vi "NOSAMSBouncerDAQold.vi"(8 "error in (no error)":errorcluster) -> (0 "error out":errorcluster, 2 "Summary Data":T3={"C12LE"=-3.412199553742333e-06, "C13LE"=5.20479903681381e-07, "C12"=7.075321622517488e-06, "C13L"=1.7362857861361653e-07, "C13H"=-1.0439441090572094e-07, "C1312"=0.009791956480809522, "Counts"=421, "LT"=47.557759786666665, "RT"=50.97312722666666, "BadBlocks"=0} {"C12LE" format="%_3e"; "C13LE" format="%_3e"; "C1312" format="%_3e"; "C12" format="%_3e"; "C13L" format="%_3e"; "C13H" format="%_3e"}, 3 "Run Average Ratios":T7={"C14Rate"=8.852393424091265, "CountErr"=0.04873701788285794, "DT"=3.415367439999997, "DTfrac"=0.06700329420269986, "C13"=144076303000.13074, "C13H/L"=-0.601251313230148, "d13C"=-128.61242295148944, "C14/13"=6.144239711705561e-11, "C12Cor"=14723744296458.893, "C13/12"=0.009791956480809522, "C14/12"=6.012324885471077e-13, "LEC13/12"=-0.15253501311508708} {"LEC13/12" format="%_4e"; "DTfrac" format="%#_3g"; "DT" format="%#_3g"; "CountErr" format="%#_3g"; "d13C" format="%_4g"; "C13/12" format="%_4e"; "C14/12" format="%_4e"; "C14/13" format="%_3e"; "C12Cor" format="%_3e"; "C13" format="%_3e"; "C13H/L" format="%#_3g"})   [LabVIEW 2011]
uses:
  RunRatios.ctl
  SummaryData.ctl
  PixieKeithleyDAQstates.ctl
  FCOffset.ctl
  BouncerParameters.ctl
  <vilib>/DAQmx/write.llb/DAQmx Write (Analog Wfm 1Chan NSamp).vi
  <vilib>/DAQmx/read.llb/DAQmx Read (Analog 1D Wfm NChan NSamp).vi
  <vilib>/DAQmx/read.llb/DAQmx Read (Counter U32 1Chan 1Samp).vi
  <vilib>/DAQmx/create/channels.llb/DAQmx Create Channel (CI-Count Edges).vi
  <vilib>/DAQmx/create/channels.llb/DAQmx Create Channel (AI-Voltage-Basic).vi
  <vilib>/DAQmx/configure/trigger.llb/DAQmx Start Trigger (Digital Edge).vi
  <vilib>/DAQmx/configure/timing.llb/DAQmx Timing (Sample Clock).vi
  <vilib>/DAQmx/create/channels.llb/DAQmx Create Channel (AO-Voltage-Basic).vi
  <vilib>/DAQmx/configure/timing.llb/DAQmx Timing (Use Waveform).vi
  <vilib>/DAQmx/create/channels.llb/DAQmx Create Channel (CO-Pulse Generation-Time).vi
  <vilib>/DAQmx/configure/timing.llb/DAQmx Timing (Implicit).vi
  <vilib>/DAQmx/miscellaneous.llb/DAQmx Fill In Error Info.vi
  Program Files/National Instruments/LabVIEW 2011/resource/objmgr/daqmx.rc
panel:
  out "Transmission":dbl format="%#_3g"
  out "C13":dbl
  out "DT Corrected Rate Ch0":dbl=8.852393424091265
  in  "Bouncer Parameters":T1={"12C Period"=0.6, "12C Delay"=400.0, "12C Voltage"=8.264999999999993, "13C Period"=0.6, "13C Delay"=200.0, "13C Voltage"=3.9999999999999996, "14C Period"=100.0, "14C Delay"=800.0, "14C Voltage"=0.41, "LE13C Period"=0.10000000000000003, "LE13C Delay"=100.0, "LE13C Voltage"=0.41, "LE12C Period"=0.20000000000000004, "LE12C Delay"=100.0, "LE12C Voltage"=4.3} {"LE12C Voltage" format="%_4f"; "LE13C Voltage" format="%_4f"; "14C Voltage" format="%_4f"; "13C Voltage" format="%_4f"; "12C Voltage" format="%_4f"}
  out "Split Cup Good":bool
  out "GetBlocktime":dbl
  out "HE 13 Ratio":waveform(dbl)(graph)={"t0"=timestamp(3425919338.3191624 s since 1904-01-01), "dt"=9.999999999999972e-06, "Y"=array[400 elements], "attributes"=variant("NI_ChannelName"=variant(string "PXI1Slot4/ai2"), "NI_UnitDescription"=variant(string "Volts"))}
  out "HE 13 SUM":waveform(dbl)(graph)={"t0"=timestamp(3425919338.3191624 s since 1904-01-01), "dt"=9.999999999999972e-06, "Y"=array[400 elements], "attributes"=variant("NI_ChannelName"=variant(string "PXI1Slot4/ai2"), "NI_UnitDescription"=variant(string "Volts"))}
  in  "low limit":dbl=1e-08
  in  "C13HLPoints":i32=10
  out "LE Currents":cluster{"C13LE":dbl, "C12LE":dbl}(graph)={"C13LE"=0.5227394525948715, "C12LE"=-3.4827548280142357}
  in  "C12":dbl=10000000.0
  in  "C13":dbl=1000000000.0
  in  "C13LE":dbl=1000000.0
  in  "C12LE":dbl=1000000.0
  out "LoopTime":u32=56
  in  "AI rate":dbl=100000.0 format="%0.2f"
  in  "AI Samples":i32=1000
  out "CH1 GDT":dbl=3.2435650133333334
  out "CH0 GDT":dbl=3.2435607466666667
  in  "FC Offset":T2={"HE 12C Offset"=0.0, "HE 13CL Offset"=0.0, "HE 13CH Offset"=0.0, "LE FC Scale"=11, "HE C12 Scale"=11, "HE C13 Scale"=18} {"HE C13 Scale" items=["500 mA/V", "200 mA/V", "100 mA/V", "50 mA/V", "20 mA/V", "10 mA/V", "5 mA/V", "2 mA/V", "1 mA/V", "500 uA/V", "200 uA/V", "100 uA/V", "50 uA/V", "20 uA/V", "10 uA/V", "5 uA/V", "2 uA/V", "1 uA/V", "500 nA/V", "200 nA/V", "100 nA/V", "50 nA/V", "20 nA/V", "10 nA/V", "5 nA/V", "2 nA/V", "1 nA/V", "500 pA/V", "200 pA/V", "100 pA/V", "50 pA/V", "20 pA/V", "10 pA/V", "5 pA/V", "2 pA/V", "1 pA/V", ""]; "HE C12 Scale" items=["500 mA/V", "200 mA/V", "100 mA/V", "50 mA/V", "20 mA/V", "10 mA/V", "5 mA/V", "2 mA/V", "1 mA/V", "500 uA/V", "200 uA/V", "100 uA/V", "50 uA/V", "20 uA/V", "10 uA/V", "5 uA/V", "2 uA/V", "1 uA/V", "500 nA/V", "200 nA/V", "100 nA/V", "50 nA/V", "20 nA/V", "10 nA/V", "5 nA/V", "2 nA/V", "1 nA/V", "500 pA/V", "200 pA/V", "100 pA/V", "50 pA/V", "20 pA/V", "10 pA/V", "5 pA/V", "2 pA/V", "1 pA/V", ""]; "LE FC Scale" items=["500 mA/V", "200 mA/V", "100 mA/V", "50 mA/V", "20 mA/V", "10 mA/V", "5 mA/V", "2 mA/V", "1 mA/V", "500 uA/V", "200 uA/V", "100 uA/V", "50 uA/V", "20 uA/V", "10 uA/V", "5 uA/V", "2 uA/V", "1 uA/V", "500 nA/V", "200 nA/V", "100 nA/V", "50 nA/V", "20 nA/V", "10 nA/V", "5 nA/V", "2 nA/V", "1 nA/V", "500 pA/V", "200 pA/V", "100 pA/V", "50 pA/V", "20 pA/V", "10 pA/V", "5 pA/V", "2 pA/V", "1 pA/V", ""]; "HE 13CH Offset" format="%.1e"; "HE 13CL Offset" format="%_2e"; "HE 12C Offset" format="%_2e"}
  out "HE 13CL Cup":waveform(dbl)(graph)={"t0"=timestamp(3425919338.3191624 s since 1904-01-01), "dt"=9.999999999999972e-06, "Y"=array[400 elements], "attributes"=variant("NI_ChannelName"=variant(string "PXI1Slot4/ai2"), "NI_UnitDescription"=variant(string "Volts"))}
  out "Bouncer":waveform(dbl)(graph)={"t0"=timestamp(3425919338.3171663 s since 1904-01-01), "dt"=9.999999999999972e-06, "Y"=array[1000 elements], "attributes"=variant("NI_ChannelName"=variant(string "PXI1Slot4/ai4"), "NI_UnitDescription"=variant(string "Volts"))}
  out "LE 13C Cup":waveform(dbl)(graph)={"t0"=timestamp(3425919338.3231645 s since 1904-01-01), "dt"=9.999999999999972e-06, "Y"=array[400 elements], "attributes"=variant("NI_ChannelName"=variant(string "PXI1Slot4/ai3"), "NI_UnitDescription"=variant(string "Volts"))}
  out "LE 12C Cup":waveform(dbl)(graph)={"t0"=timestamp(3425919338.3191648 s since 1904-01-01), "dt"=9.999999999999972e-06, "Y"=array[400 elements], "attributes"=variant("NI_ChannelName"=variant(string "PXI1Slot4/ai3"), "NI_UnitDescription"=variant(string "Volts"))}
  out "HE 13CH Cup":waveform(dbl)(graph)={"t0"=timestamp(3425919338.3191605 s since 1904-01-01), "dt"=9.999999999999972e-06, "Y"=array[400 elements], "attributes"=variant("NI_ChannelName"=variant(string "PXI1Slot4/ai1"), "NI_UnitDescription"=variant(string "Volts"))}
  out "HE 12C Cup":waveform(dbl)(graph)={"t0"=timestamp(3425919338.3171587 s since 1904-01-01), "dt"=9.999999999999972e-06, "Y"=[-0.00044240412530680836, -0.0012475330618199733, -0.00044240412530680836, 4.0673236898795524e-05, -0.000603429912659012, -0.00028137833792978424, 0.0003627248118268677, 0.0005237505993282573, 0.0002016990243503863, -0.000603429912659012, -0.00012035255052792213, -0.00028137833792978424, -0.00044240412530680836, -0.0010865072745668758, -0.0007644556999864127, -0.0007644556999864127, 0.0003627248118268677, 0.0002016990243503863, 0.0003627248118268677, -0.00044240412530680836, -0.00028137833792978424, 0.0006847763868545727, 0.0008458021744058315, -0.00012035255052792213, -0.00012035255052792213, -0.000603429912659012, 0.0018119569002381763, 0.0006847763868545727, 0.0006847763868545727, -0.000603429912659012, 0.0005237505993282573, -0.00012035255052792213, 0.0006847763868545727, -0.00044240412530680836, 0.0024560600512941624, 0.016787355268375024, 0.04883148805412984, 0.08393511228220728, 0.10502949274489624, 0.10390231209407401, 0.08570639611485263, 0.06428996459086032, 0.04979764282936263, 0.0502807202173878, 0.059942268035882144, 0.07314638357140049, 0.08329100907135802, 0.0860284477212322, 0.08248588005856013, 0.0733074093719574, 0.06557817098196769, 0.06155252601651977, 0.06461201618844556, 0.0696038159674263, 0.07411253837523522, 0.07701100279387124, 0.07540074478219393, 0.07298535777087642, 0.07073099656697797, 0.06847663536946497, 0.06912073856810563, 0.06895971276839691, 0.07137509976743812, 0.0733074093719574, 0.07362946097316983, 0.07298535777087642, 0.07282433197038517, 0.07008689336703908, 0.0696038159674263, 0.07185817716812601, 0.07137509976743812, 0.07105304816714282, 0.07201920296842067, 0.070247919166975, 0.07137509976743812, 0.07121407396727417, 0.07040894496694343, 0.07073099656697797, 0.07137509976743812, 0.07105304816714282, 0.07169715136786403, 0.07282433197038517, 0.07056997076694442, 0.07137509976743812, 0.07185817716812601, 0.07137509976743812, 0.07266330616992672, 0.07137509976743812, 0.07218022876874806, 0.07282433197038517, 0.07298535777087642, 0.07266330616992672, 0.07234125456910818, 0.07234125456910818, 0.07105304816714282, 0.07250228036950107, 0.07169715136786403, 0.0733074093719574, 0.07314638357140049, 0.07234125456910818, 0.07250228036950107, 0.07234125456910818, 0.07234125456910818, 0.06445099038963699, 0.07266330616992672, 0.07201920296842067, 0.07121407396727417, 0.07427356417598957, 0.07153612556763475, 0.07218022876874806, 0.07250228036950107, 0.07153612556763475, 0.06992586756713566, 0.07169715136786403, 0.07169715136786403, 0.07185817716812601, 0.07282433197038517, 0.07234125456910818, 0.07234125456910818, 0.07073099656697797, 0.07185817716812601, 0.07234125456910818, 0.07282433197038517, 0.07282433197038517, 0.07121407396727417, 0.07169715136786403, 0.07218022876874806, 0.07153612556763475, 0.07234125456910818, 0.07298535777087642, 0.07266330616992672, 0.07218022876874806, 0.07218022876874806, 0.07169715136786403, 0.07201920296842067, 0.07250228036950107, 0.07298535777087642, 0.07298535777087642, 0.07250228036950107, 0.07282433197038517, 0.07153612556763475, 0.07201920296842067, 0.07298535777087642, 0.07185817716812601, 0.07169715136786403, 0.07201920296842067, 0.07250228036950107, 0.07234125456910818, 0.07266330616992672, 0.07218022876874806, 0.07169715136786403, 0.07137509976743812, 0.07169715136786403, 0.07185817716812601, 0.07234125456910818, 0.07169715136786403, 0.07185817716812601, 0.07314638357140049, 0.07282433197038517, 0.07266330616992672, 0.07266330616992672, 0.07169715136786403, 0.07362946097316983, 0.07040894496694343, 0.07056997076694442, 0.07169715136786403, 0.07314638357140049, 0.07218022876874806, 0.07266330616992672, 0.07218022876874806, 0.07137509976743812, 0.07282433197038517, 0.07169715136786403, 0.07185817716812601, 0.07298535777087642, 0.07185817716812601, 0.070247919166975, 0.07201920296842067, 0.07201920296842067, 0.07201920296842067, 0.0708920223670441, 0.07234125456910818, 0.0696038159674263, 0.07153612556763475, 0.07201920296842067, 0.07073099656697797, 0.07169715136786403, 0.07121407396727417, 0.07201920296842067, 0.07185817716812601, 0.07121407396727417, 0.07153612556763475, 0.07121407396727417, 0.0708920223670441, 0.0708920223670441, 0.07266330616992672, 0.07185817716812601, 0.07218022876874806, 0.07121407396727417, 0.07137509976743812], "attributes"=variant("NI_ChannelName"=variant(string "PXI1Slot4/ai0"), "NI_UnitDescription"=variant(string "Volts"))}
  out "C13LE":dbl=5.251065316204094e-07 format="%_4g"
  out "C12LE":dbl=-3.801022287660527e-06 format="%_4g"
  out "DT Corrected Rate Ch1":dbl=8.852393424091265
  out "SCA Rate":dbl=0.0009971750496192643
  out "SCA Counts":u32=450
  out "CH1 SFDT":dbl=0.17075989333333333 format="%#_2f"
  out "CH0 SFDT":dbl=1.17997632 format="%#_2f"
  in  "Mode":enum16{"Tuning", "Run", "Manual"}(ring)
  out "Block Spectrum":u32[][](graph) caption="ADC Spectrum"
  out "RunningAverages":T3={"C12LE"=-3.4827548280142356e-06, "C13LE"=5.227394525948715e-07, "C12"=7.01043378332938e-06, "C13L"=1.7393577894450557e-07, "C13H"=-1.0546050382879386e-07, "C1312"=0.009770783306647468, "Counts"=3, "LT"=0.3472770133333327, "RT"=0.34875175999999897, "BadBlocks"=0} {"C12LE" format="%_3e"; "C13LE" format="%_3e"; "C1312" format="%_3e"; "C12" format="%_3e"; "C13L" format="%_3e"; "C13H" format="%_3e"}
  out "Elapsed Time":dbl=451274.829 format="%#_6f"
  out "element":T4=enum."Idle"
  in  "Stop":bool
  in  "Stop DAQ":bool
  in  "Run Parameters":T5={"Block time (s)"=0.1, "Max Runtime (s)"=100000.0, "Max Counts"=100000, "C12 Limit"=-1.0, "Max BadBlocks"=100} {"Block time (s)" min=0.0 max=100.0 step=0.1}
  out "Acquiring":bool
  in  "StartDAQ":bool
  in  "Logfile":string="May13.txt"
  in  "Log File Path":path=path "C:/DAQ Logs"
  out "Good Block":bool=TRUE
  out "Currents & Counts":cluster{"C14Rate":dbl, "C12":dbl, dbl}(graph)={"C14Rate"=8.638636836928967, "C12"=68.47527511571171, 70.1043378332938}
  out "Ratios":T6(graph)={"C14/12"=6.012324885471077e-13, "C14/12"=5.921452435682224e-13, "d13C"=-128.61242295148944, "d13C"=-130.4966266821389}
  out "13C H/L":dbl(knob)=-0.6063186336288013 scale=0.0..2.0 scale format="%#_3g"
  out "Currents":cluster{dbl, dbl}(knob)={7.01043378332938e-06, 6.847527511571172e-08} scale=0.0..0.0001 scale format="%#_1e"
  out "Moving Average Ratios":T7={"C14Rate"=8.638636836928967, "CountErr"=0.5773502691896257, "DT"=0.001474746666666249, "DTfrac"=0.004228642936930995, "C13"=142497047515.79608, "C13H/L"=-0.6063186336288013, "d13C"=-130.4966266821389, "C14/13"=6.062326895559963e-11, "C12Cor"=14588712703108.44, "C13/12"=0.009770783306647468, "C14/12"=5.921452435682224e-13, "LEC13/12"=-0.15009366964051332} {"LEC13/12" format="%_4e"; "DTfrac" format="%#_3g"; "DT" format="%#_3g"; "CountErr" format="%#_3g"; "d13C" format="%_4g"; "C13/12" format="%_4e"; "C14/12" format="%_4e"; "C14/13" format="%_3e"; "C12Cor" format="%_3e"; "C13" format="%_3e"; "C13H/L" format="%#_3g"}
  in  "CountPoints":i32=5 min=1
  in  "CurPoints":i32=5 min=1
  out "C12":dbl=7.1950767003945815e-06 format="%_4g"
  out "C13L":dbl=1.7373499980027144e-07 format="%_4g"
  out "C13H":dbl=-1.0672666958653134e-07 format="%_4g"
  out "Run time [s]":dbl=50.97312722666666 format="%_6g"
  out "Ch1 LT":dbl=50.97208469333333
  out "Ch1 Counts":u32=421
  out "Ch1 Rate":dbl=8.259422829827143
  out "Ch0 LT":dbl=50.973052159999995
  out "Ch0 Counts":u32=423
  out "Ch0 Rate":dbl=8.298502484650902
  # "Currents (A)"
  # "13C x100"
  # "Counts"
  # "Livetime"
  # "Rate"
  # "SFDT"
  # "GDT"
  # "Cor Rate"
  # "Ch 0"
  # "Ch1"
  # "SCA"
  # "ms"
  # "us"
  # "kV"
  # "ms"
  # "us"
  # "kV"
  # "ms"
  # "us"
  # "kV"
  # "ms"
  # "us"
  # "kV"
  # "ms"
  # "us"
  # "kV"
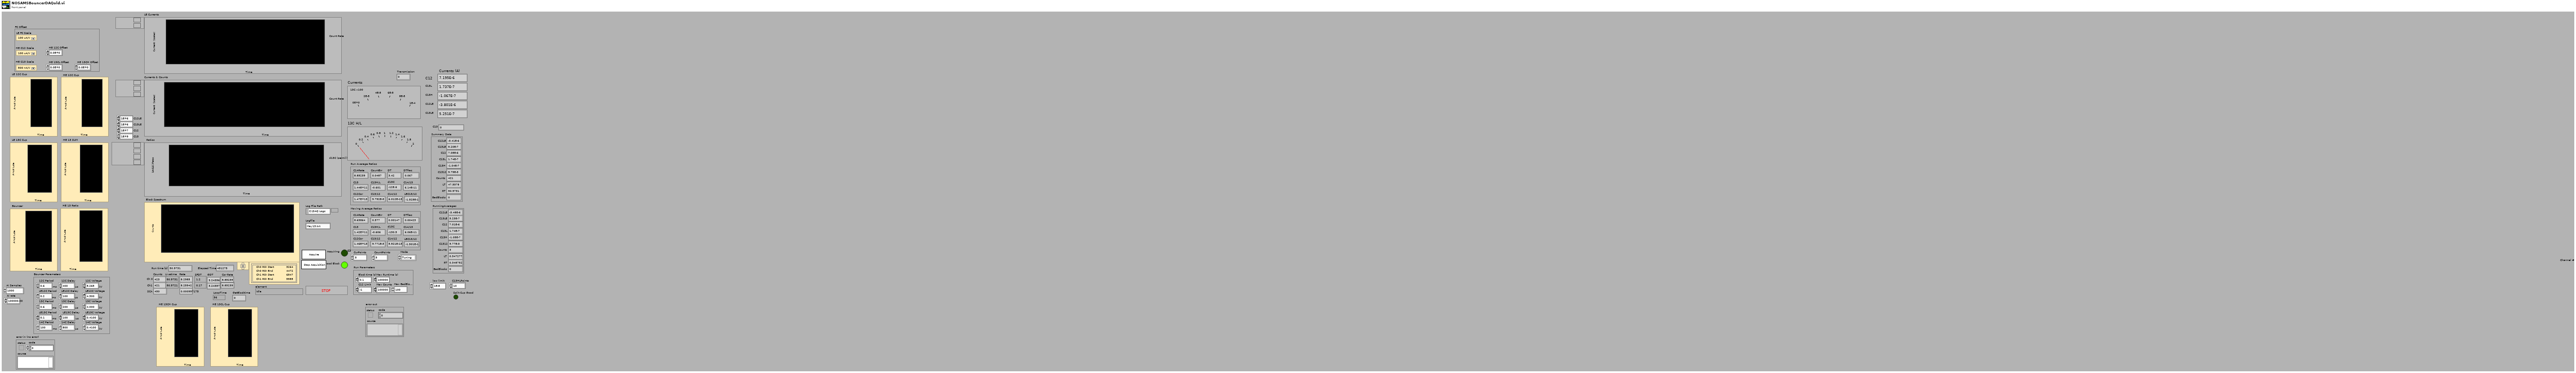
[diagram p1: front panel]
types:
  T1 = typedef "BouncerParameters.ctl" = cluster{"12C Period":dbl, "12C Delay":dbl, "12C Voltage":dbl, "13C Period":dbl, "13C Delay":dbl, "13C Voltage":dbl, "14C Period":dbl, "14C Delay":dbl, "14C Voltage":dbl, "LE13C Period":dbl, "LE13C Delay":dbl, "LE13C Voltage":dbl, "LE12C Period":dbl, "LE12C Delay":dbl, "LE12C Voltage":dbl}
  T2 = typedef "FCOffset.ctl" = cluster{"HE 12C Offset":dbl, "HE 13CL Offset":dbl, "HE 13CH Offset":dbl, "LE FC Scale":u16, "HE C12 Scale":u16, "HE C13 Scale":u16}
  T3 = typedef "SummaryData.ctl" = cluster{"C12LE":dbl, "C13LE":dbl, "C12":dbl, "C13L":dbl, "C13H":dbl, "C1312":dbl, "Counts":u32, "LT":dbl, "RT":dbl, "BadBlocks":u8}
  T4 = typedef "PixieKeithleyDAQstates.ctl" = enum16{"Initialize", "Restart Bouncer", "Idle", "Start Run", "Wait", "Get Block", "Check Data", "Check Run", "Analyse and Display", "Stop DAQ", "Log Data", "Stop"}
  T5 = cluster{"Block time (s)":dbl, "Max Runtime (s)":dbl, "Max Counts":u32, "C12 Limit":dbl, "Max BadBlocks":u8}
  T6 = cluster{"C14/12":dbl, "C14/12":dbl, "d13C":dbl, "d13C":dbl}
  T7 = typedef "RunRatios.ctl" = cluster{"C14Rate":dbl, "CountErr":dbl, "DT":dbl, "DTfrac":dbl, "C13":dbl, "C13H/L":dbl, "d13C":dbl, "C14/13":dbl, "C12Cor":dbl, "C13/12":dbl, "C14/12":dbl, "LEC13/12":dbl}
  T8 = typedef "BlockData.ctl" = cluster{"LE C12":dbl[], "LE C13":dbl[], "C12":dbl[], "C13L":dbl[], "C13H":dbl[], "C1312":dbl[], "Counts":u32[], "LT":dbl[], "RT":dbl[]}
  T9 = typedef "LVCursorListTypeDef.ctl" = cluster{"Name":string, "Color":u32, "Style":u8, "Point Style":u8, "Name Visible":bool, "Allow Drag":bool, "Cursor Mode":u32, "Plot":i32, "Index":i32, "Position":cluster{"X":dbl, "Y":dbl}, "X Scale":u32, "Y Scale":u32, "Watch Plots":i32[], "Watch All Plots":bool, "Plot Area":i32, "Label Offset":cluster{"X":dbl, "Y":dbl}}[]
  T10 = cluster{"Ch0 Counts":u32, "Ch0 Rate":dbl, "Ch1 Counts":u32, "Ch1 Rate":dbl}
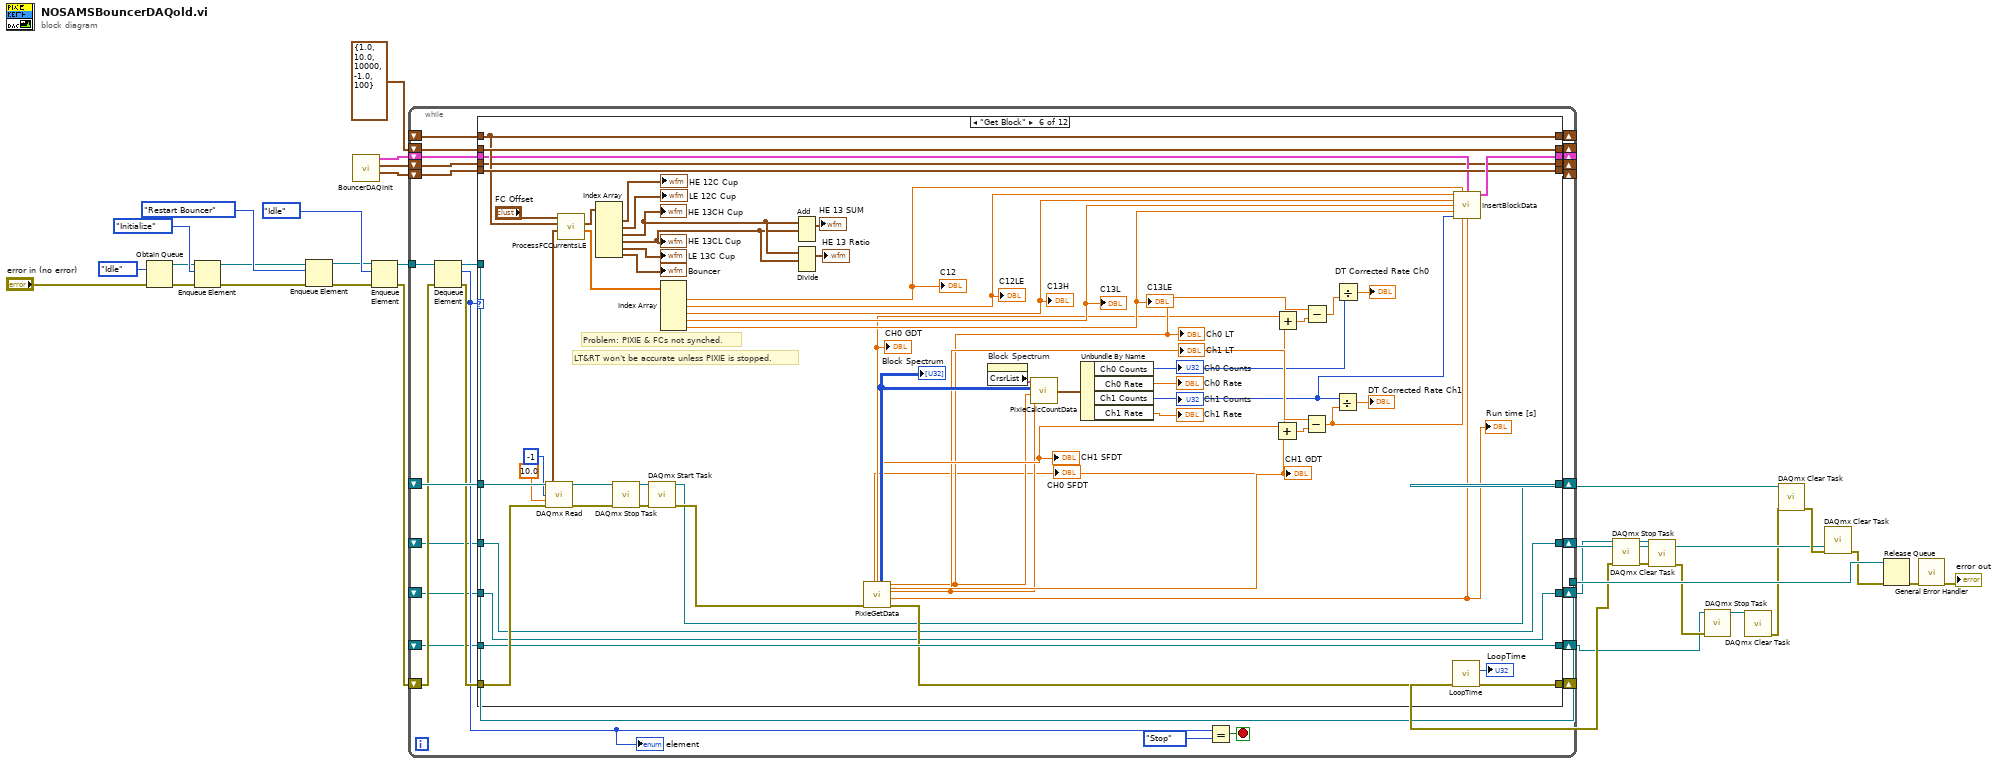
[diagram p0: block diagram]
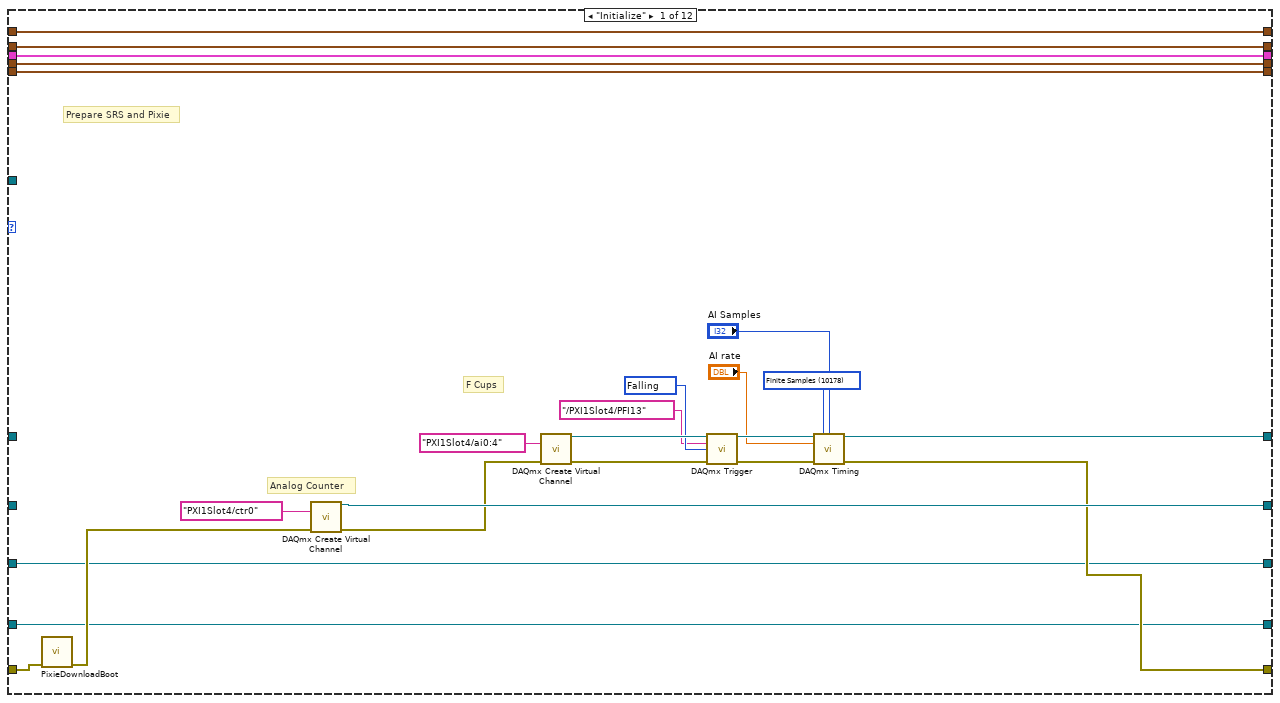
[diagram p2: hidden frame]
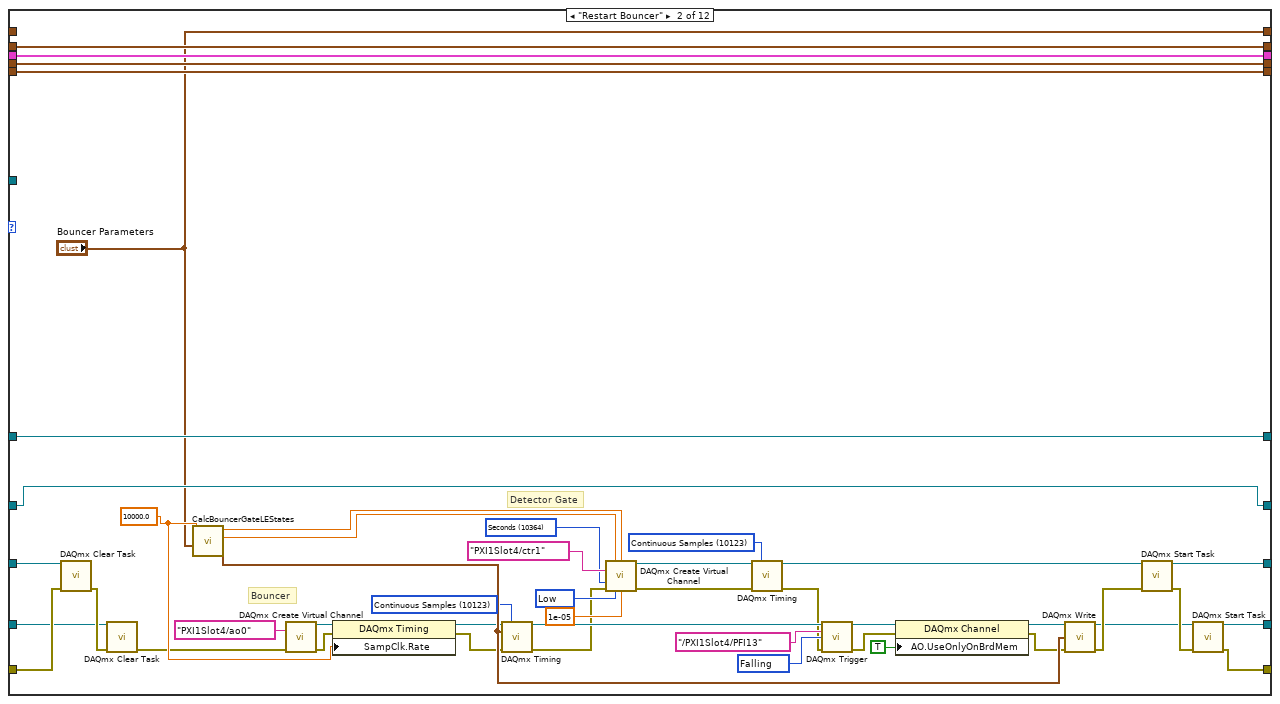
[diagram p3: hidden frame]
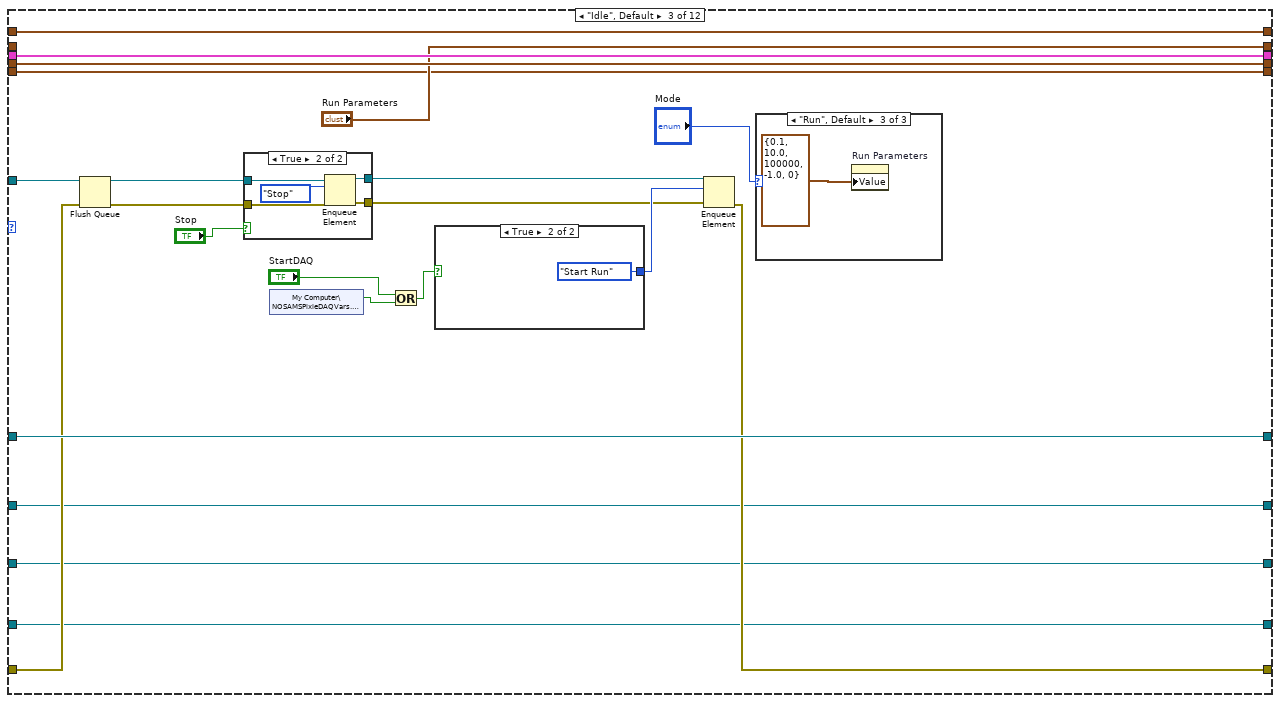
[diagram p4: hidden frame]
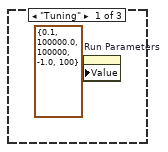
[diagram p5: hidden frame]
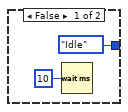
[diagram p8: hidden frame]
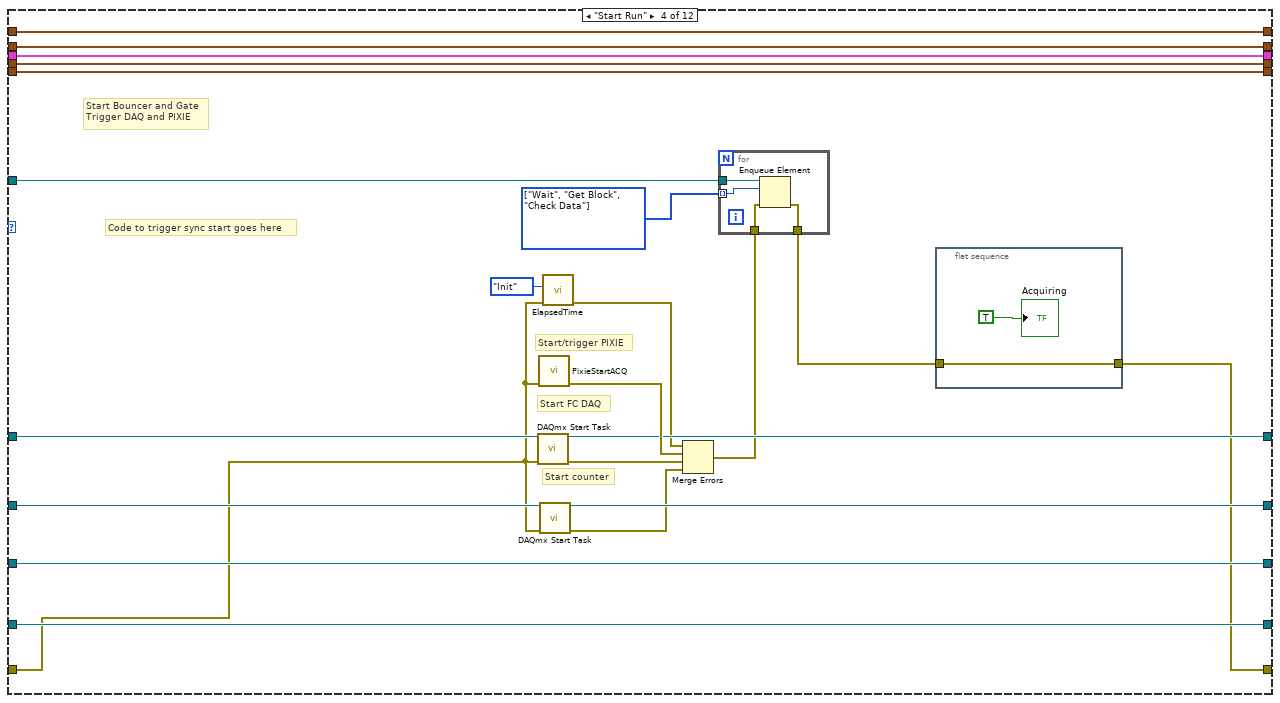
[diagram p9: hidden frame]
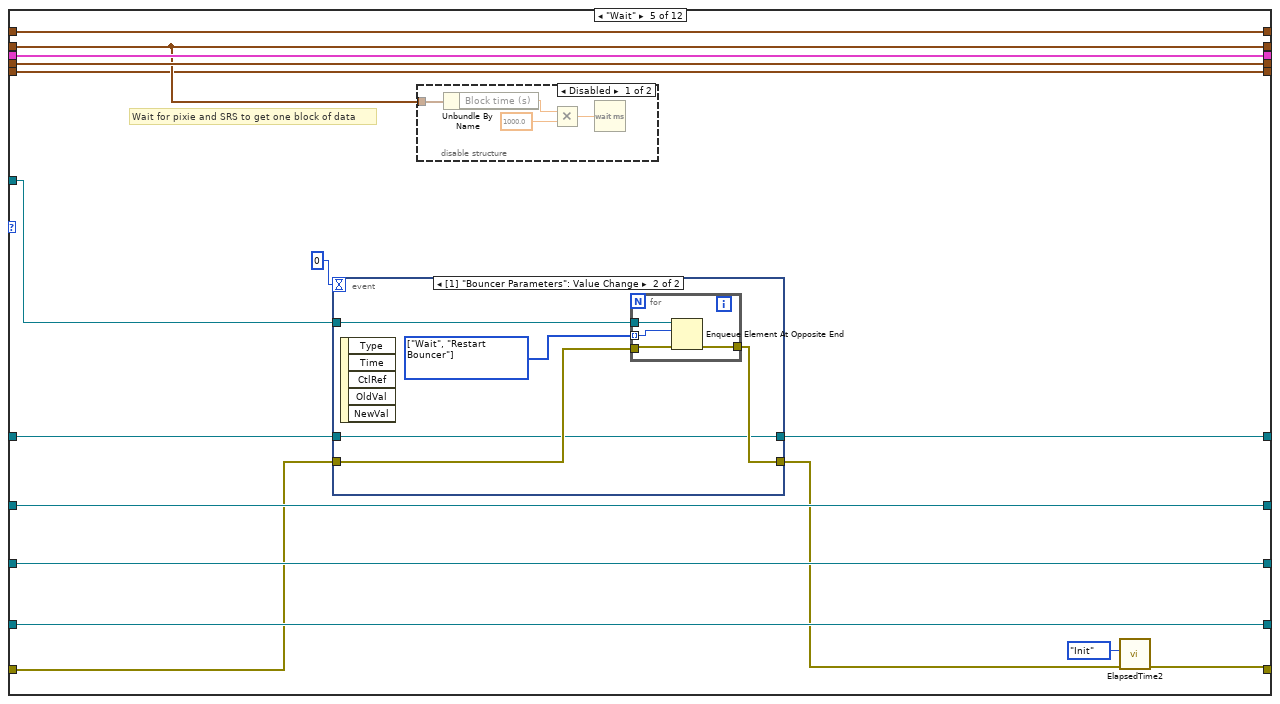
[diagram p10: hidden frame]
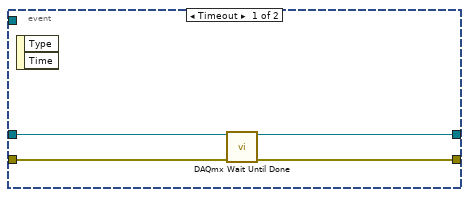
[diagram p11: hidden frame]
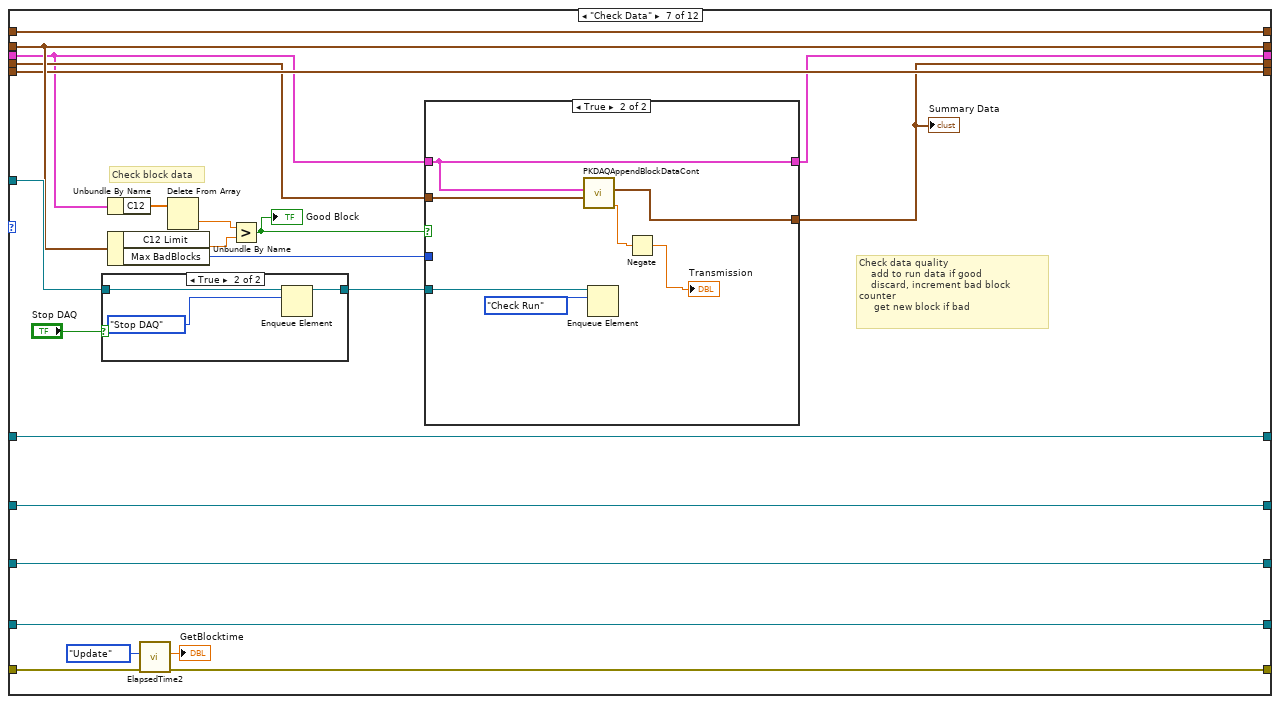
[diagram p13: hidden frame]
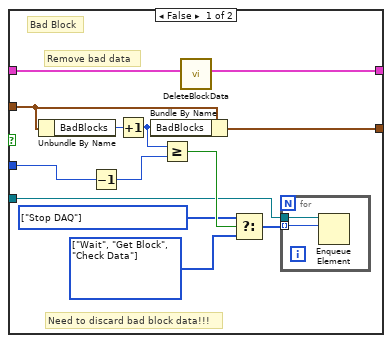
[diagram p15: hidden frame]
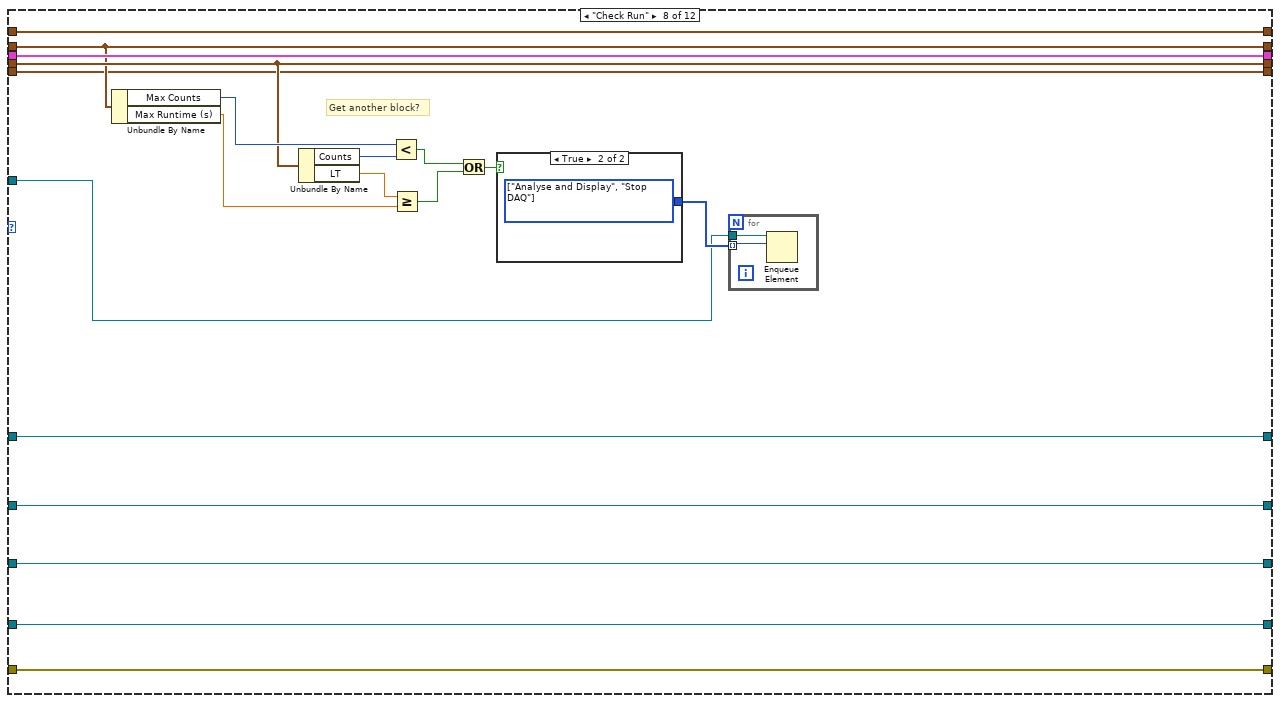
[diagram p16: hidden frame]
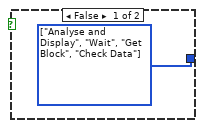
[diagram p17: hidden frame]
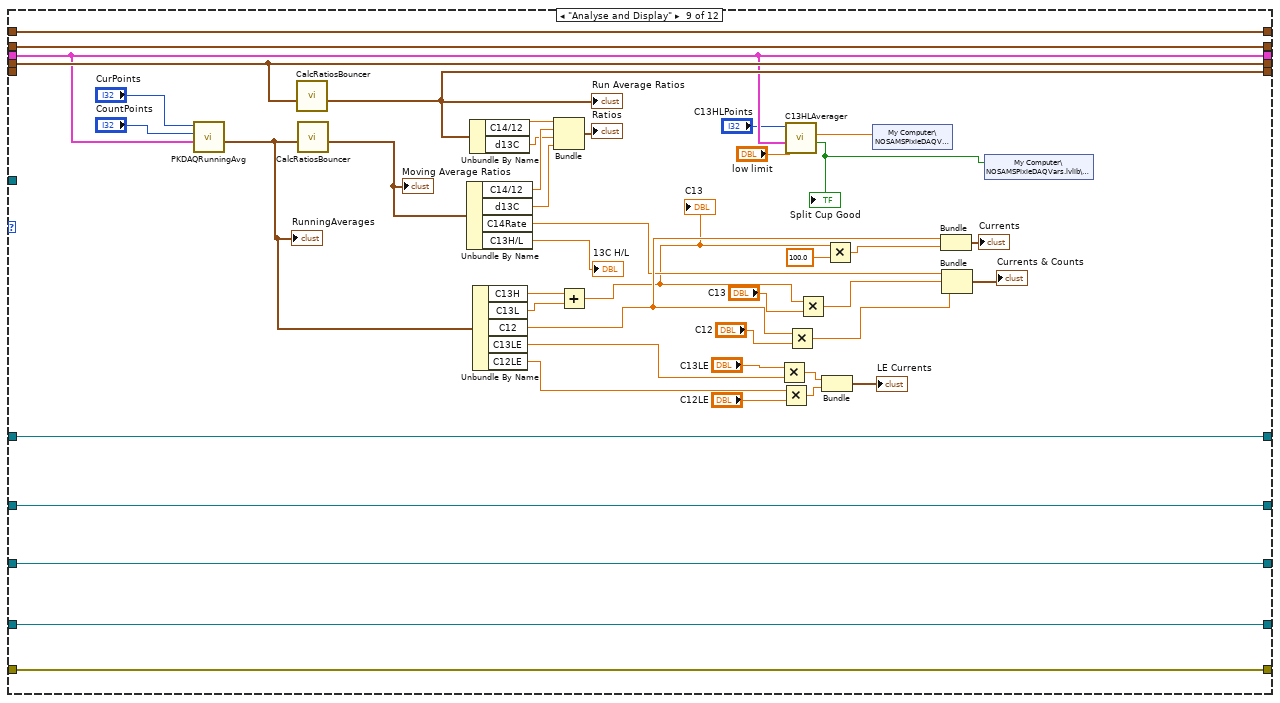
[diagram p18: hidden frame]
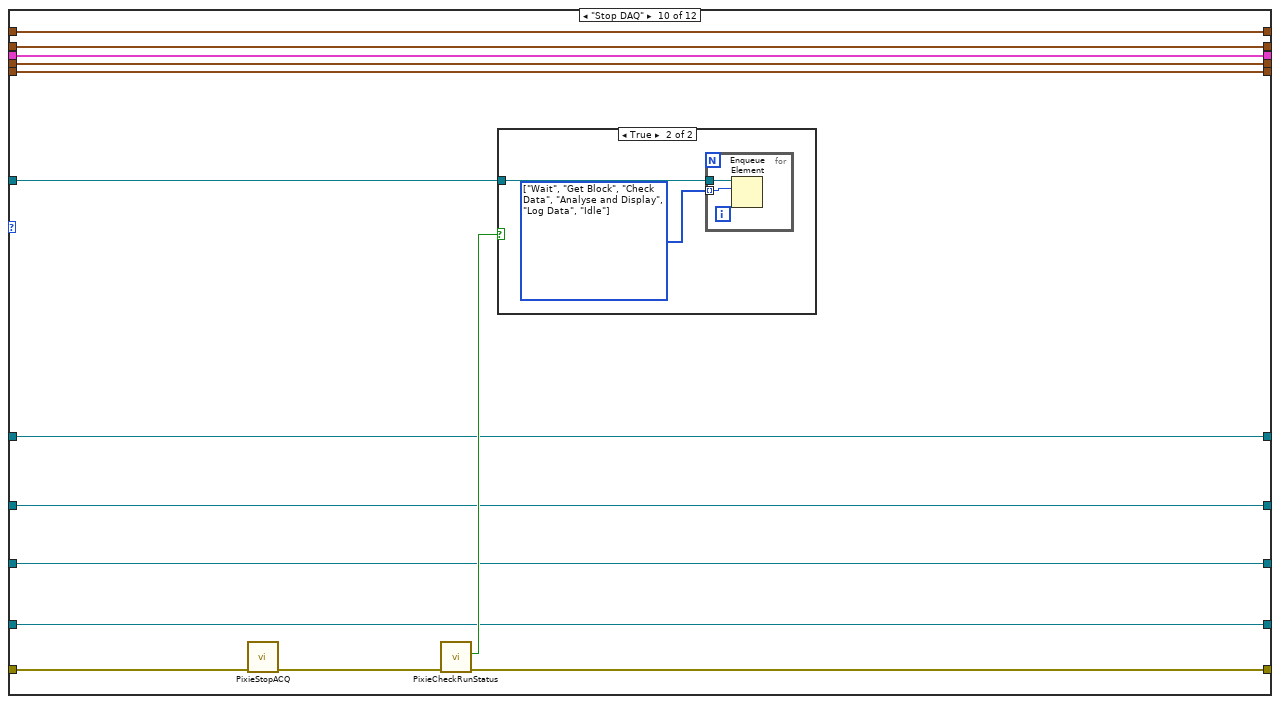
[diagram p19: hidden frame]
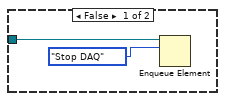
[diagram p20: hidden frame]
diagram:
  n1 = Obtain Queue(element data type=PixieKeithleyDAQstates."Idle" ("Next State"), error in (no error)="error in (no error)") -> (queue out=w24:refnum<queue>, error out=w23:errorcluster)  [unwired: 2 in, 2 out]
  n2 = Enqueue Element(queue=w24, element=PixieKeithleyDAQstates."Initialize", error in (no error)=w23) -> (queue out=w10:refnum<queue>, error out=w12:errorcluster)  [unwired: 2 out]
  n3 = Enqueue Element(queue=w10, element=PixieKeithleyDAQstates."Restart Bouncer", error in (no error)=w12) -> (queue out=w9:refnum<queue>, error out=w11:errorcluster)  [unwired: 2 out]
  n4 = call "BouncerDAQinit.vi"() -> ("Run Ratios"=w19:T7, "Summary Data"=w18:T3, "Block Data"=w17:T8)  [unwired: 2 in, 7 out]
  n5 = Enqueue Element(queue=w9, element=PixieKeithleyDAQstates."Idle", error in (no error)=w11) -> (queue out=w29:refnum<queue>, error out=w28:errorcluster)  [unwired: 2 out]
  n6 = while {
    shift-right: [w54] -> _
    shift-left: w17 -> [w55]
    shift-right: [w52] -> _
    shift-left: w18 -> [w53]
    shift-right: [w33] -> w32
    shift-left: _ -> [w51]
    shift-right: [w56] -> w5
    shift-left: w28 -> [w48]
    tunnel: w29 -> [w50]
    tunnel: [w47] -> w26
    shift-right: [w46] -> _
    shift-left: T5 {"Block time (s)"=1.0, "Max Runtime (s)"=10.0, "Max Counts"=10000, "C12 Limit"=-1.0, "Max BadBlocks"=100} ("Run Parameters 2") -> [w45]
    shift-right: [w42] -> _
    shift-left: w19 -> [w43]
    shift-right: [w41] -> w14
    shift-left: _ -> [w40]
    shift-right: [w39] -> w2
    shift-left: _ -> [w36]
    shift-right: [w38] -> w7
    shift-left: _ -> [w37]
    shift-right: [w35] -> _
    shift-left: _ -> [w34]
    stop <- w58 stop-if-true
    n7 = Dequeue Element(queue=w50, error in (no error)=w48) -> (queue out=w47:refnum<queue>, element=w44:T4, error out=w49:errorcluster)  [unwired: 2 out]
    "element" <- w44
    n8 = case shown="\"Get Block\"" w44 {
      tunnel: [w62 w90 w143 w163 w191 w234 w283 w350 w398 w404 w444 w468] -> w56
      tunnel: w49 -> [w78 w99 w145 w165 w196 w266 w284 w350 w398 w406 w432 w468]
      tunnel: w55 -> [w82 w95 w150 w184 w206 w246 w288 w346 w362 w412 _ w473]
      tunnel: [w82 w95 w150 w184 w206 w279 w287 w346 w362 w412 w438 w473] -> w54
      tunnel: w53 -> [w81 w94 w149 w183 w205 w244 w290 w343 w383 w411 w422 w472]
      tunnel: [w81 w94 w149 w183 w205 w244 w289 w343 w383 w411 w439 w472] -> w52
      tunnel: w45 -> [w77 w96 _ w174 w204 w274 w297 w339 w388 w405 w446 w467]
      tunnel: w51 -> [_ w92 w148 w180 w198 w282 w304 w347 w397 w407 w448 w469]
      tunnel: w47 -> [_ _ w147 w176 w194 _ w299 w337 _ w408 _ w470]
      tunnel: [w77 w96 "Run Parameters" w174 w204 w274 w297 w339 w388 w405 w446 w467] -> w46
      tunnel: w43 -> [w76 w93 w136 w172 w203 w273 w295 w336 _ w403 w421 w466]
      tunnel: [w76 w93 w136 w172 w203 w273 w295 w336 w387 w403 w440 w466] -> w42
      tunnel: [w74 w91 w135 w170 w202 w225 w294 w335 w386 w402 w434 w465] -> w41
      tunnel: w40 -> [_ w91 w135 w171 w202 w225 w294 w335 w386 w402 w437 w465]
      tunnel: [w60 w84 w133 w167 w200 w265 w292 w333 w384 w400 w425 w463] -> w39
      tunnel: [w61 w87 w134 w168 w201 w226 w293 w334 w385 w401 w426 w464] -> w38
      tunnel: w37 -> [w61 w97 w134 w168 w201 w226 w293 w334 w385 w401 w426 w464]
      tunnel: w36 -> [w60 w98 w133 w167 w200 w265 w292 w333 w384 w400 w425 w463]
      tunnel: [w59 "Bouncer Parameters" w132 w166 w199 w254 w291 w332 w382 w399 w424 w462] -> w35
      tunnel: w34 -> [w59 _ w132 w166 w199 w254 w291 w332 w382 w399 w424 w462]
      tunnel: [w63 w92 w148 w179 w197 w224 w304 w347 w397 w407 w447 w469] -> w33
      frame "Initialize" {
        w68 = 10171 items=["Rising"=10280, "Falling"=10171] ("edge")
        w79 = 10178 items=["Finite Samples"=10178, "Continuous Samples"=10123] ("sample mode")
        # "Analog Counter"
        # "F Cups"
        # "Prepare SRS and Pixie"
        n9 = call "PixieDownloadBoot.vi"("error in (no error)"=w78) -> ("error out"=w66:errorcluster)  [unwired: 5 in, 5 out]
        n10 = call-poly <vilib>:"DAQmx Create Virtual Channel.vi"("counter"=tag "PXI1Slot4/ctr0" ("Counter(s)"), "error in"=w66) -> ("task out"=w74:refnum<k21>, "error out"=w73:errorcluster)  [unwired: 5 in, 7 out]
        n11 = call-poly <vilib>:"DAQmx Create Virtual Channel.vi"("physical channels"=tag "PXI1Slot4/ai0:4", "error in"=w73) -> ("task out"=w72:refnum<k21>, "error out"=w70:errorcluster)  [unwired: 7 in, 5 out]
        n12 = call-poly <vilib>:"DAQmx Trigger.vi"("task/channels in"=w72, "source"=tag "/PXI1Slot4/PFI13", "edge"=w68, "error in"=w70) -> ("task out"=w71:refnum<k21>, "error out"=w69:errorcluster)  [unwired: 10 in]
        n13 = call-poly <vilib>:"DAQmx Timing.vi"("task/channels in"=w71, "sample mode"=w79, "samples per channel"="AI Samples", "rate"="AI rate", "error in"=w69) -> ("task out"=w63:refnum<k21>, "error out"=w62:errorcluster)  [unwired: 2 in, 7 out]
      }
      frame "Restart Bouncer" {
        w115 = 10171 items=["Rising"=10280, "Falling"=10171] ("edge")
        w113 = 10123 items=["Finite Samples"=10178, "Continuous Samples"=10123] ("sample mode")
        w110 = 10123 items=["Finite Samples"=10178, "Continuous Samples"=10123, "Hardware Timed Single Point"=12522] ("sample mode")
        w105 = 10214 items=["High"=10192, "Low"=10214] ("idle state")
        w106 = 10364 items=["Seconds"=10364] ("units")
        w128 = 10000.0 ("rate")
        # "Bouncer"
        # "Detector Gate"
        n14 = call <vilib>:"DAQmx Clear Task.vi"("task in"=w97, "error in"=w99) -> ("error out"=w100:errorcluster)  [unwired: 13 in]
        n15 = call <vilib>:"DAQmx Clear Task.vi"("task in"=w98, "error in"=w100) -> ("error out"=w101:errorcluster)  [unwired: 13 in]
        n16 = call "CalcBouncerGateLEStates.vi"("Bouncer Settings"="Bouncer Parameters", "SampClk.Rate"=w128) -> ("Bouncer Waveform"=w127:waveform(dbl), "High time"=w112:dbl, "low time"=w111:dbl)  [unwired: 7 in]
        n17 = call-poly <vilib>:"DAQmx Create Virtual Channel.vi"("physical channels"=tag "PXI1Slot4/ao0", "error in"=w101) -> ("task out"=w123:refnum<k21>, "error out"=w122:errorcluster)  [unwired: 7 in, 5 out]
        n18 = property class="DAQmx Timing"(reference=w123, error in=w122, "SampClk.Rate"=w128) -> (reference out=w124:refnum<k21>, error out=w125:errorcluster)
        n19 = call-poly <vilib>:"DAQmx Timing.vi"("task/channels in"=w124, "sample mode"=w113, "waveform"=w127, "error in"=w125) -> ("task out"=w114:refnum<k21>, "error out"=w103:errorcluster)  [unwired: 10 out]
        n20 = call-poly <vilib>:"DAQmx Create Virtual Channel.vi"("high time"=w112, "low time"=w111, "counter"=tag "PXI1Slot4/ctr1", "units"=w106, "error in"=w103, "idle state"=w105, "initial delay"=1e-05) -> ("task out"=w109:refnum<k21>, "error out"=w108:errorcluster)  [unwired: 2 in, 5 out]
        n21 = call-poly <vilib>:"DAQmx Timing.vi"("task/channels in"=w109, "sample mode"=w110, "error in"=w108) -> ("task out"=w88:refnum<k21>, "error out"=w102:errorcluster)  [unwired: 1 in, 10 out]
        n22 = call-poly <vilib>:"DAQmx Trigger.vi"("task/channels in"=w114, "source"=tag "/PXI1Slot4/PFI13", "edge"=w115, "error in"=w102) -> ("task out"=w118:refnum<k21>, "error out"=w120:errorcluster)  [unwired: 10 out]
        n23 = property class="DAQmx Channel"(reference=w118, error in=w120, "AO.UseOnlyOnBrdMem"=TRUE) -> (reference out=w119:refnum<k21>, error out=w121:errorcluster)
        n24 = call-poly <vilib>:"DAQmx Write.vi"("task/channels in"=w119, "data"=w127, "error in"=w121) -> ("task out"=w85:refnum<k21>, "error out"=w86:errorcluster)  [unwired: 1 in, 10 out]
        n25 = call <vilib>:"DAQmx Start Task.vi"("task/channels in"=w88, "error in"=w86) -> ("task out"=w87:refnum<k21>, "error out"=w89:errorcluster)  [unwired: 12 in]
        n26 = call <vilib>:"DAQmx Start Task.vi"("task/channels in"=w85, "error in"=w89) -> ("task out"=w84:refnum<k21>, "error out"=w90:errorcluster)  [unwired: 12 in]
      }
      frame "Idle", Default {
        n27 = Flush Queue(queue=w147, error in (no error)=w145) -> (queue out=w141:refnum<queue>, error out=w139:errorcluster)  [unwired: 1 out]
        n28 = case shown="True" "Stop" {
          tunnel: w141 -> [w154 w159]
          tunnel: [w154 w158] -> w140
          tunnel: w139 -> [w153 w157]
          tunnel: [w153 w156] -> w138
          frame False {
          }
          frame True {
            n29 = Enqueue Element(queue=w159, element=PixieKeithleyDAQstates."Stop", error in (no error)=w157) -> (queue out=w158:refnum<queue>, error out=w156:errorcluster)  [unwired: 2 out]
          }
        }
        n30 = shared-variable "My Computer\\NOSAMSPixieDAQVars.lvlib\\StartDAQ"() -> (w131:bool)  [unwired: 1 in, 1 out]
        n31 = Or(x="StartDAQ", y=w131) -> (x .or. y?=w129:bool)
        n32 = case shown="True" w129 {
          tunnel: [PixieKeithleyDAQstates."Idle" ("element") PixieKeithleyDAQstates."Start Run" ("element")] -> w146
          frame False {
            n33 = Wait (ms)(milliseconds to wait=u32 10) -> ()  [unwired: 1 out]
          }
          frame True {
          }
        }
        n34 = Enqueue Element(queue=w140, element=w146, error in (no error)=w138) -> (error out=w143:errorcluster)  [unwired: 3 out]
        n35 = case shown="\"Run\", Default" "Mode" {
          frame "Tuning" {
            n36 = property on="Run Parameters" class="Clust (strict)"("Value"=T5 {"Block time (s)"=0.1, "Max Runtime (s)"=100000.0, "Max Counts"=100000, "C12 Limit"=-1.0, "Max BadBlocks"=100} ("Run Parameters")) -> ()  [unwired: 2 in, 2 out]
          }
          frame "Manual" {
          }
          frame "Run", Default {
            n37 = property on="Run Parameters" class="Clust (strict)"("Value"=T5 {"Block time (s)"=0.1, "Max Runtime (s)"=10.0, "Max Counts"=100000, "C12 Limit"=-1.0, "Max BadBlocks"=0} ("Run Parameters")) -> ()  [unwired: 2 in, 2 out]
          }
        }
      }
      frame "Start Run" {
        w173 = T4[] [enum."Wait", enum."Get Block", enum."Check Data"] items=["Initialize", "Restart Bouncer", "Idle", "Start Run", "Wait", "Get Block", "Check Data", "Check Run", "Analyse and Display", "Stop DAQ", "Log Data", "Stop"]
        # "Start Bouncer and Gate\nTrigger DAQ and PIXIE"
        # "Start counter"
        # "Code to trigger sync start goes here"
        # "Start/trigger PIXIE"
        # "Start FC DAQ"
        n38 = call <vilib>:"DAQmx Start Task.vi"("task/channels in"=w180, "error in"=w165) -> ("task out"=w179:refnum<k21>, "error out"=w182:errorcluster)  [unwired: 12 out]
        n39 = call "PixieStartACQ.vi"("error in (no error)"=w165) -> ("error out"=w181:errorcluster)  [unwired: 2 in, 8 out]
        n40 = call <vilib>:"DAQmx Start Task.vi"("task/channels in"=w171, "error in"=w165) -> ("task out"=w170:refnum<k21>, "error out"=w169:errorcluster)  [unwired: 12 out]
        n41 = call "ElapsedTime.vi"("error in (no error)"=w165, "Mode (Update)"=enum16{"Update", "Init"}."Init") -> ("error out"=w178:errorcluster)  [unwired: 9 out]
        n42 = Merge Errors(w178, w181, w182, w169) -> (w175:errorcluster)
        n43 = for {
          tunnel: w176 -> [w190]
          tunnel: w175 -> [w189]
          tunnel: [w188] -> w164
          tunnel: w173 -> [w187] mode=indexing
          n44 = Enqueue Element(queue=w190, element=w187, error in (no error)=w189) -> (error out=w188:errorcluster)  [unwired: 3 out]
        }
        n45 = flat-sequence {
          tunnel: w164 -> [w185]
          tunnel: [w185] -> w163
          frame #0 {
            "Acquiring" <- TRUE
          }
        }
      }
      frame "Wait" {
        # "Wait for pixie and SRS to get one block of data"
        n46 = event shown="[1] \"Bouncer Parameters\": Value Change" {
          selector: _ -> [_ _]
          dyn-events: _ -> [_ _]
          timeout: 0 -> [_ _]
          tunnel: w198 -> [w210 w212]
          tunnel: [w209 w212] -> w197
          tunnel: w196 -> [w208 w214]
          tunnel: [w207 w213] -> w192
          tunnel: w194 -> [_ w211]
          event Timeout {
            n47 = event-data() -> ()  [unwired: 1 in, 2 out]
            n48 = call <vilib>:"DAQmx Wait Until Done.vi"("task/channels in"=w210, "error in"=w208) -> ("task out"=w209:refnum<k21>, "error out"=w207:errorcluster)  [unwired: 12 in]
          }
          event Value Change {
            w215 = T4[] [enum."Wait", enum."Restart Bouncer"] items=["Initialize", "Restart Bouncer", "Idle", "Start Run", "Wait", "Get Block", "Check Data", "Check Run", "Analyse and Display", "Stop DAQ", "Log Data", "Stop"]
            n49 = event-data() -> ()  [unwired: 1 in, 5 out]
            n50 = for {
              tunnel: w211 -> [w219]
              tunnel: w214 -> [w218]
              tunnel: [w217] -> w213
              tunnel: w215 -> [w216] mode=indexing
              n51 = Enqueue Element At Opposite End(queue=w219, element=w216, error in (no error)=w218) -> (error out=w217:errorcluster)  [unwired: 1 in, 2 out]
            }
          }
        }
        n52 = disable-structure shown="Disabled" {
          disable-tunnel: w204 -> [w220 _]
          frame Disabled {
            n53 = Unbundle By Name(w220) -> ("Block time (s)"=w222:dbl)
            n54 = Multiply(x=w222, y=1000.0) -> (x*y=w221:dbl)
            n55 = Wait (ms)(milliseconds to wait=w221) -> ()  [unwired: 1 out]
          }
          frame Enabled {
          }
        }
        n56 = call "ElapsedTime2.vi"("error in (no error)"=w192, "Mode (Update)"=enum16{"Update", "Init"}."Init") -> ("error out"=w191:errorcluster)  [unwired: 8 in, 1 out]
      }
      frame "Get Block" {
        # "LT&RT won't be accurate unless PIXIE is stopped."
        # "Problem: PIXIE & FCs not synched."
        n57 = call-poly <vilib>:"DAQmx Read.vi"("task/channels in"=w282, "number of samples per channel"=-1, "timeout"=10.0, "error in"=w266) -> ("task out"=w253:refnum<k21>, "data"=w270:waveform(dbl)[], "error out"=w237:errorcluster)  [unwired: 9 out]
        n58 = call "ProcessFCCurrentsLE.vi"("FC Data"=w270, "Bouncer Settings"=w254, "FC Offset"="FC Offset") -> ("Mean Currents"=w268:dbl[], "Output Waveforms"=w269:waveform(dbl)[])  [unwired: 7 in]
        n59 = Index Array(array=w269) -> (element #1=→"HE 12C Cup":waveform(dbl), element #2=→"LE 12C Cup":waveform(dbl), element #3=w240:waveform(dbl), element #4=w239:waveform(dbl), element #5=→"LE 13C Cup":waveform(dbl), element #6=→"Bouncer":waveform(dbl))  [unwired: 6 in]
        "HE 13CL Cup" <- w239
        "HE 13CH Cup" <- w240
        n60 = call <vilib>:"DAQmx Stop Task.vi"("task/channels in"=w253, "error in"=w237) -> ("task out"=w252:refnum<k21>, "error out"=w251:errorcluster)  [unwired: 12 in]
        n61 = call <vilib>:"DAQmx Start Task.vi"("task/channels in"=w252, "error in"=w251) -> ("task out"=w224:refnum<k21>, "error out"=w236:errorcluster)  [unwired: 12 in]
        n62 = Index Array(array=w268) -> (element #1=w247:dbl, element #2=w249:dbl, element #3=w264:dbl, element #4=w263:dbl, element #5=w248:dbl)  [unwired: 5 in]
        "C13H" <- w264
        "C13L" <- w263
        "C12" <- w247
        "C12LE" <- w249
        "C13LE" <- w248
        n63 = Add(1:w239, 2:w240) -> (0:→"HE 13 SUM":waveform(dbl))  [unwired: 1 in, 1 out]
        n64 = Divide(1:w239, 2:w240) -> (0:→"HE 13 Ratio":waveform(dbl))  [unwired: 1 in, 1 out]
        n65 = call "PixieGetData.vi"("error IO"=w236) -> ("error out"=w235:errorcluster, "Run time [s]"=w271:dbl, "CH1 LT"=w259:dbl, "CH0 LT"=w229:dbl, "CH1 SFDT"=w260:dbl, "Histogram Data"=w278:u32[][], "CH0 SFDT"=w227:dbl, "CH1 GDT"=w261:dbl, "CH0 GDT"=w228:dbl)  [unwired: 2 in]
        "Block Spectrum" <- w278
        "Ch0 LT" <- w229
        "Ch1 LT" <- w259
        "Run time [s]" <- w271
        "CH0 SFDT" <- w227
        "CH1 SFDT" <- w260
        "CH0 GDT" <- w228
        "CH1 GDT" <- w261
        n66 = property on="Block Spectrum" class="WFGraph (strict)"() -> ("CrsrList"=w277:T9)  [unwired: 2 in, 2 out]
        n67 = call "PixieCalcCountData.vi"("CrsrList"=w277, "Histogram Data"=w278, "CH0 LT"=w229, "CH1 LT"=w259) -> ("Count Data"=w276:T10)  [unwired: 1 in]
        n68 = Unbundle By Name(w276) -> ("Ch0 Counts"=w230:u32, "Ch0 Rate"=→"Ch0 Rate":dbl, "Ch1 Counts"=w245:u32, "Ch1 Rate"=→"Ch1 Rate":dbl)
        "Ch0 Counts" <- w230
        "Ch1 Counts" <- w245
        n69 = Add(x=w260, y=w261) -> (x+y=w262:dbl)
        n70 = Add(x=w228, y=w227) -> (x+y=w233:dbl)
        n71 = Subtract(x=w259, y=w262) -> (x-y=w243:dbl)
        n72 = Subtract(x=w229, y=w233) -> (x-y=w231:dbl)
        n73 = Divide(x=w245, y=w243) -> (x/y=→"DT Corrected Rate Ch1":dbl)
        n74 = Divide(x=w230, y=w231) -> (x/y=→"DT Corrected Rate Ch0":dbl)
        n75 = call "LoopTime.vi"("error in (no error)"=w235) -> ("error out"=w234:errorcluster, "LoopTime"=→"LoopTime":u32)  [unwired: 9 in]
        n76 = call "InsertBlockData.vi"("C12LE"=w249, "C12"=w247, "Block Data In"=w246, "C13H"=w264, "C13L"=w263, "C13LE"=w248, "Counts"=w245, "LT"=w243, "RT"=w271) -> ("Block Data Out"=w279:T8)  [unwired: 6 in]
      }
      frame "Check Data" {
        # "Check block data"
        # "Check data quality\n    add to run data if good\n    discard, increment bad block counter\n     get new block if bad"
        n77 = case shown="True" "Stop DAQ" {
          tunnel: w299 -> [w306 w309]
          tunnel: [w306 w308] -> w298
          frame False {
          }
          frame True {
            n78 = Enqueue Element(queue=w309, element=PixieKeithleyDAQstates."Stop DAQ" ("Next State")) -> (queue out=w308:refnum<queue>)  [unwired: 1 in, 3 out]
          }
        }
        n79 = Unbundle By Name(w288) -> ("C12"=w303:dbl[])
        n80 = Unbundle By Name(w297) -> ("C12 Limit"=w305:dbl, "Max BadBlocks"=w300:u8)
        n81 = call "ElapsedTime2.vi"("error in (no error)"=w284, "Mode (Update)"=enum16{"Update", "Init"}."Update") -> ("error out"=w283:errorcluster, "Elapsed Time"=→"GetBlocktime":dbl)  [unwired: 8 in]
        n82 = Delete From Array(array=w303) -> (deleted portion=w302:dbl)  [unwired: 2 in, 1 out]
        n83 = Greater?(x=w302, y=w305) -> (0:w301:bool)
        "Good Block" <- w301
        n84 = case shown="True" w301 {
          tunnel: [w321 w328] -> w289
          tunnel: w290 -> [w322 w329]
          tunnel: w288 -> [w311 w327]
          tunnel: w300 -> [w320 _]
          tunnel: w298 -> [w318 w331]
          tunnel: [w310 w327] -> w287
          frame False {
            w315 = T4[] [enum."Wait", enum."Get Block", enum."Check Data"] items=["Initialize", "Restart Bouncer", "Idle", "Start Run", "Wait", "Get Block", "Check Data", "Check Run", "Analyse and Display", "Stop DAQ", "Log Data", "Stop"]
            w317 = T4[] [enum."Stop DAQ"] items=["Initialize", "Restart Bouncer", "Idle", "Start Run", "Wait", "Get Block", "Check Data", "Check Run", "Analyse and Display", "Stop DAQ", "Log Data", "Stop"]
            # "Remove bad data"
            # "Need to discard bad block data!!!"
            # "Bad Block"
            n85 = Unbundle By Name(w322) -> ("BadBlocks"=w314:u8)
            n86 = Decrement(x=w320) -> (x-1=w313:u8)
            n87 = Increment(x=w314) -> (x+1=w312:u8)
            n88 = Bundle By Name(cluster=w322, "BadBlocks"=w312) -> (w321:T3)
            n89 = Greater Or Equal?(x=w312, y=w313) -> (x >= y?=w319:bool)
            n90 = call "DeleteBlockData.vi"("Block Data In"=w311) -> ("Block Data Out"=w310:T8)  [unwired: 10 in]
            n91 = Select(t=w317, s=w319, f=w315) -> (s? t:f=w316:T4[])
            n92 = for {
              tunnel: w316 -> [w324] mode=indexing
              tunnel: w318 -> [w323]
              n93 = Enqueue Element(queue=w323, element=w324) -> ()  [unwired: 1 in, 4 out]
            }
          }
          frame True {
            n94 = call "PKDAQAppendBlockDataCont.vi"("Run Summary"=w329, "Block Data"=w327) -> ("Transmission"=w326:dbl, "Run Summary Out"=w328:T3)  [unwired: 8 out]
            n95 = Enqueue Element(queue=w331, element=PixieKeithleyDAQstates."Check Run") -> ()  [unwired: 1 in, 4 out]
            n96 = Negate(x=w326) -> (-x=→"Transmission":dbl)
          }
        }
        "Summary Data" <- w289
      }
      frame "Check Run" {
        # "Get another block?"
        n97 = Unbundle By Name(w339) -> ("Max Counts"=w349:u32, "Max Runtime (s)"=w348:dbl)
        n98 = Unbundle By Name(w343) -> ("Counts"=w345:u32, "LT"=w344:dbl)
        n99 = Less?(x=w349, y=w345) -> (x < y?=w341:bool)
        n100 = Greater Or Equal?(x=w344, y=w348) -> (x >= y?=w340:bool)
        n101 = Or(x=w341, y=w340) -> (x .or. y?=w342:bool)
        n102 = case shown="True" w342 {
          tunnel: [w353 w354] -> w338
          frame False {
            w353 = T4[] [enum."Analyse and Display", enum."Wait", enum."Get Block", enum."Check Data"] items=["Initialize", "Restart Bouncer", "Idle", "Start Run", "Wait", "Get Block", "Check Data", "Check Run", "Analyse and Display", "Stop DAQ", "Log Data", "Stop"]
          }
          frame True {
            w354 = T4[] [enum."Analyse and Display", enum."Stop DAQ"] items=["Initialize", "Restart Bouncer", "Idle", "Start Run", "Wait", "Get Block", "Check Data", "Check Run", "Analyse and Display", "Stop DAQ", "Log Data", "Stop"]
          }
        }
        n103 = for {
          tunnel: w337 -> [w352]
          tunnel: w338 -> [w351] mode=indexing
          n104 = Enqueue Element(queue=w352, element=w351) -> ()  [unwired: 1 in, 4 out]
        }
      }
      frame "Analyse and Display" {
        n105 = call "PKDAQRunningAvg.vi"("Block Data"=w362, "CountPoints"="CountPoints", "CurPoints"="CurPoints") -> ("RunningAverages"=w376:T3)  [unwired: 8 out]
        "RunningAverages" <- w376
        n106 = call "CalcRatiosBouncer.vi"("Run Summary"=w383) -> ("Run Ratios"=w387:T7)  [unwired: 10 out]
        "Run Average Ratios" <- w387
        n107 = call "CalcRatiosBouncer.vi"("Run Summary"=w376) -> ("Run Ratios"=w394:T7)  [unwired: 10 out]
        "Moving Average Ratios" <- w394
        n108 = Unbundle By Name(w394) -> ("C14/12"=w392:dbl, "d13C"=w389:dbl, "C14Rate"=w364:dbl, "C13H/L"=→"13C H/L":dbl)
        n109 = Unbundle By Name(w387) -> ("C14/12"=w393:dbl, "d13C"=w390:dbl)
        n110 = Unbundle By Name(w376) -> ("C13H"=w374:dbl, "C13L"=w373:dbl, "C12"=w367:dbl, "C13LE"=w371:dbl, "C12LE"=w368:dbl)
        n111 = Bundle("C14/12"=w393, "C14/12"=w392, "d13C"=w390, "d13C"=w389) -> (→"Ratios":T6)  [unwired: 1 out]
        n112 = Add(x=w374, y=w373) -> (x+y=w355:dbl)
        "C13" <- w355
        n113 = Multiply(x="C13LE", y=w371) -> (x*y=w370:dbl)
        n114 = Multiply(x=w368, y="C12LE") -> (x*y=w369:dbl)
        n115 = call "C13HLAverager.vi"("Block Data"=w362, "low limit"="low limit", "CurPoints"="C13HLPoints") -> ("13CCurrent"=w358:bool, "C13HL"=w360:dbl)  [unwired: 7 in]
        "Split Cup Good" <- w358
        n116 = Multiply(x=w367, y="C12") -> (x*y=w366:dbl)
        n117 = Multiply(x=w355, y="C13") -> (x*y=w365:dbl)
        n118 = Bundle(w370, w369) -> (→"LE Currents":cluster{dbl, dbl})  [unwired: 1 out]
        n119 = Multiply(x=w355, y=100.0) -> (x*y=w356:dbl)
        n120 = shared-variable "My Computer\\NOSAMSPixieDAQVars.lvlib\\C13HL"(w360) -> ()  [unwired: 1 in, 1 out]
        n121 = Bundle("C12"=w367, w356) -> (→"Currents":cluster{"C12":dbl, dbl})  [unwired: 1 out]
        n122 = Bundle("C14Rate"=w364, w365, w366) -> (→"Currents & Counts":cluster{"C14Rate":dbl, dbl, dbl})  [unwired: 1 out]
        n123 = shared-variable "My Computer\\NOSAMSPixieDAQVars.lvlib\\C13HLGood"(w358) -> ()  [unwired: 1 in, 1 out]
      }
      frame "Stop DAQ" {
        n124 = call "PixieStopACQ.vi"("error in (no error)"=w406) -> ("error out"=w410:errorcluster)  [unwired: 10 out]
        n125 = call "PixieCheckRunStatus.vi"("error in (no error)"=w410) -> ("error out"=w404:errorcluster, "run finished"=w409:bool)  [unwired: 1 in, 8 out]
        n126 = case shown="True" w409 {
          tunnel: w408 -> [w414 w416]
          frame False {
            n127 = Enqueue Element(queue=w414, element=PixieKeithleyDAQstates."Stop DAQ" ("Next State")) -> ()  [unwired: 1 in, 4 out]
          }
          frame True {
            w415 = T4[] [enum."Wait", enum."Get Block", enum."Check Data", enum."Analyse and Display", enum."Log Data", enum."Idle"] items=["Initialize", "Restart Bouncer", "Idle", "Start Run", "Wait", "Get Block", "Check Data", "Check Run", "Analyse and Display", "Stop DAQ", "Log Data", "Stop"]
            n128 = for {
              tunnel: w416 -> [w418]
              tunnel: w415 -> [w417] mode=indexing
              n129 = Enqueue Element(queue=w418, element=w417) -> ()  [unwired: 1 in, 4 out]
            }
          }
        }
      }
      frame "Log Data" {
        # "Add data to status file and return here?"
        # "Return to DAQ Control\nData if good run\nError condition if bad"
        n130 = call "ElapsedTime.vi"("error in (no error)"=w432) -> ("error out"=w431:errorcluster, "Elapsed Time"=w430:dbl)  [unwired: 1 in, 8 out]
        "Elapsed Time" <- w430
        n131 = call-poly <vilib>:"DAQmx Read.vi"("task/channels in"=w437, "error in"=w431) -> ("task out"=w436:refnum<k21>, "data"=w429:u32, "error out"=w435:errorcluster)  [unwired: 1 in, 10 out]
        "SCA Counts" <- w429
        n132 = flat-sequence {
          tunnel: w422 -> [w452]
          tunnel: w421 -> [w451]
          tunnel: w420 -> [w450]
          tunnel: [w450] -> w419
          frame #0 {
            n133 = Unbundle By Name(w451) -> ("d13C"=w457:dbl, "C14/12"=w456:dbl)
            n134 = Unbundle By Name(w452) -> ("C12"=w461:dbl, "C13L"=w455:dbl, "C13H"=w453:dbl, "Counts"=w460:u32, "LT"=w459:dbl, "RT"=w458:dbl)
            n135 = shared-variable "My Computer\\NOSAMSPixieDAQVars.lvlib\\C12Cur"(w461) -> ()  [unwired: 2 out]
            n136 = shared-variable "My Computer\\NOSAMSPixieDAQVars.lvlib\\C13LCur"(w455) -> ()  [unwired: 2 out]
            n137 = shared-variable "My Computer\\NOSAMSPixieDAQVars.lvlib\\C13HCur"(w453) -> ()  [unwired: 2 out]
            n138 = shared-variable "My Computer\\NOSAMSPixieDAQVars.lvlib\\Counts"(w460) -> ()  [unwired: 2 out]
            n139 = shared-variable "My Computer\\NOSAMSPixieDAQVars.lvlib\\Livetime"(w459) -> ()  [unwired: 2 out]
            n140 = shared-variable "My Computer\\NOSAMSPixieDAQVars.lvlib\\Runtime"(w458) -> ()  [unwired: 2 out]
            n141 = shared-variable "My Computer\\NOSAMSPixieDAQVars.lvlib\\d13C"(w457) -> ()  [unwired: 1 in, 1 out]
            n142 = shared-variable "My Computer\\NOSAMSPixieDAQVars.lvlib\\C1412"(w456) -> ()  [unwired: 1 in, 1 out]
            n143 = Add(x=w455, y=w453) -> (x+y=w454:dbl)
            n144 = shared-variable "My Computer\\NOSAMSPixieDAQVars.lvlib\\C13"(w454) -> ()  [unwired: 1 in, 1 out]
          }
        }
        n145 = call <vilib>:"DAQmx Stop Task.vi"("task/channels in"=w436, "error in"=w435) -> ("task out"=w434:refnum<k21>, "error out"=w433:errorcluster)  [unwired: 12 out]
        n146 = call <vilib>:"DAQmx Stop Task.vi"("task/channels in"=w448, "error in"=w433) -> ("task out"=w447:refnum<k21>, "error out"=w420:errorcluster)  [unwired: 12 out]
        n147 = Divide(x=w429, y=w430) -> (x/y=→"SCA Rate":dbl)
        n148 = Build Path(base path="Log File Path", name or relative path="Logfile") -> (appended path=w441:path)
        n149 = call "LogSummary.vi"("error in (no error)"=w419, "Run Ratios"=w421, "Run Summary"=w422, "Log File Path"=w441) -> ("error out"=w449:errorcluster)  [unwired: 7 out]
        n150 = call "BouncerDAQinit.vi"("error in (no error)"=w449) -> ("error out"=w427:errorcluster, "Run Ratios"=w440:T7, "Summary Data"=w439:T3, "Block Data"=w438:T8)  [unwired: 1 in, 6 out]
        n151 = shared-variable "My Computer\\NOSAMSPixieDAQVars.lvlib\\C13HLGood"(FALSE ("C13HLGood")) -> ()  [unwired: 1 in, 1 out]
        n152 = shared-variable "My Computer\\NOSAMSPixieDAQVars.lvlib\\Acquiring"(FALSE ("Acquire"), error in=w427) -> (error out=w444:errorcluster)
      }
      frame "Stop" {
        n153 = Enqueue Element(queue=w470, element=PixieKeithleyDAQstates."Stop" ("Next State")) -> ()  [unwired: 1 in, 4 out]
      }
    }
    n154 = Equal?(x=w44, y=PixieKeithleyDAQstates."Stop" ("States")) -> (x = y?=w58:bool)
  }
  n155 = call <vilib>:"DAQmx Stop Task.vi"("task/channels in"=w7, "error in"=w5) -> ("task out"=w6:refnum<k21>, "error out"=w4:errorcluster)  [unwired: 12 out]
  n156 = call <vilib>:"DAQmx Clear Task.vi"("task in"=w6, "error in"=w4) -> ("error out"=w3:errorcluster)  [unwired: 13 in]
  n157 = call <vilib>:"DAQmx Stop Task.vi"("task/channels in"=w2, "error in"=w3) -> ("task out"=w1:refnum<k21>)  [unwired: 13 out]
  n158 = call <vilib>:"DAQmx Clear Task.vi"("task in"=w1) -> ("error out"=w8:errorcluster)  [unwired: 14 in]
  n159 = call <vilib>:"DAQmx Clear Task.vi"("task in"=w32, "error in"=w8) -> ("error out"=w16:errorcluster)  [unwired: 13 out]
  n160 = call <vilib>:"DAQmx Clear Task.vi"("task in"=w14, "error in"=w16) -> ("error out"=w15:errorcluster)  [unwired: 13 out]
  n161 = Release Queue(queue=w26, error in (no error)=w15) -> (error out=w21:errorcluster)  [unwired: 3 out]
  n162 = call <vilib>:"General Error Handler.vi"("error in (no error)"=w21) -> ("error out"=→"error out":errorcluster)  [unwired: 1 in, 13 out]
